vi "Read.vi"(0 "System Interface in":refnum<class "System Interface.lvclass">, 11 "Error In":errorcluster) -> (4 "System Interface out":refnum<class "System Interface.lvclass">, 6 "Process Data":T1, 15 "Error Out":errorcluster)   [LabVIEW 2020, in "ADAS_Data_Type_Template.lvlib"]
uses:
  ADAS_Data_Type_Template.lvlib
  <vilib>/FlexLogger/SDK/PluginSDK.lvlibp/PEFClasses/SDK/System Interface/System Interface.lvclass
  Process Data.ctl
  4520f411-daba-4182-bc35-841ea590f987.vi
  4520f411-daba-4182-bc35-841ea590f987.vi/2c215e65-9050-4251-816a-3dfe657ae557.vi
  4520f411-daba-4182-bc35-841ea590f987.vi/4e5fc8e4-156f-454f-acee-b5bf5bc57c95.vi
  4520f411-daba-4182-bc35-841ea590f987.vi/2c215e65-9050-4251-816a-3dfe657ae557.vi/7bf3da57-5b1d-4b21-896d-7766261ce726.vi
  4520f411-daba-4182-bc35-841ea590f987.vi/2c215e65-9050-4251-816a-3dfe657ae557.vi/3b588064-68fc-43f0-9f28-230c287437e0.vi
  <vilib>/ADAS Record/IODataPEF/Error/Error_SetError.vi
  <vilib>/ADAS Record/IODataPEF/Error/Error_CheckAndSetDllError.vi
  <vilib>/ADAS Record/CustomData/_Custom_RegisterType.vi
  <vilib>/ADAS Record/IODataPEF/Error/ErrorMgr.vi
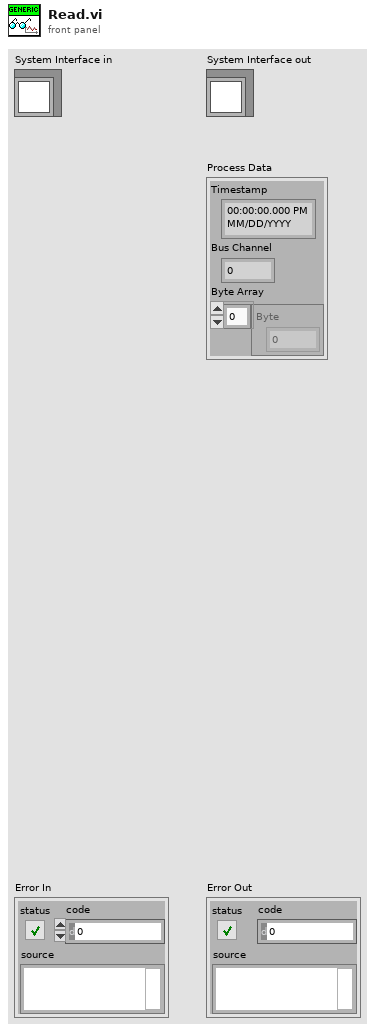
[diagram p1: front panel]
types:
  T1 = typedef "ADAS_Data_Type_Template.lvlib/Process Data.ctl" = cluster{"Timestamp":timestamp, "Bus Channel":u16, "Byte Array":u8[]}
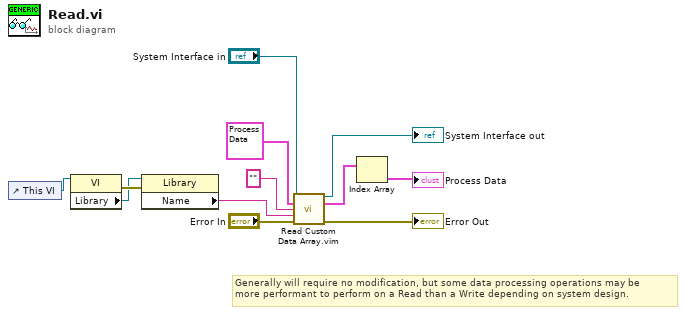
[diagram p0: block diagram]
diagram:
  # "Generally will require no modification, but some data processing operations may be\nmore performant to perform on a Read than a Write depending on system design."
  n1 = control-ref of="This VI"() -> (w4:refnum<vi>)
  n2 = property class="VI"(reference=w4) -> (error out=w3:errorcluster, "Library"=w2:refnum<vi>)  [unwired: 1 in, 1 out]
  n3 = property class="Library"(reference=w2, error in=w3) -> ("Name"=w1:string)  [unwired: 2 out]
  n4 = call "Read Custom Data Array.vim"("System Interface"="System Interface in", "Data Element Type"=T1 {"Timestamp"=timestamp(0 s since 1904-01-01), "Bus Channel"=0, "Byte Array"=[]} ("Process Data"), "Metadata Element Type"="" ("appended array"), "Type"=w1, "error in (no error)"="Error In") -> ("System Interface out"=→"System Interface out":refnum<class "System Interface.lvclass">, "Data Array"=w5:T1[], "error out"=→"Error Out":errorcluster)  [unwired: 5 in, 3 out]
  n5 = Index Array(array=w5) -> (element=→"Process Data":T1)  [unwired: 1 in]
